vi "Property Dialog.vi"(6 "Control Ref Queue":T12, 7 "Multiplot Representation":T13, 8 "error in (no error)":errorcluster, 11 "2D Compass.lvclass in":refnum<class "2D Compass.lvclass">) -> (0 "error out":errorcluster, 3 "2D Compass.lvclass out":refnum<class "2D Compass.lvclass">, 4 "Cancel?":bool)   [LabVIEW 2020, in "2D Compass.lvclass"]
uses:
  <vilib>/Math Plots/2D Math Plots/2D Compass/2D Compass/2D Compass.lvclass
  e:/builds/penguin/labview/branches/2020/dev/dist/vi.lib/Math Plots/2D Math Plots/2D Plot/2D Plot/2D Plot.lvclass
  <vilib>/Math Plots/2D Math Plots/2D Plot/Action String/2DMathPlot Ctrl Act Queue.ctl
  <vilib>/Math Plots/2D Math Plots/2D Plot/Action String/2DMathPlot Ctrl Act Cluster.ctl
  <vilib>/Math Plots/2D Math Plots/2D Plot/Action String/2DMathPlot State Class.ctl
  <vilib>/Math Plots/2D Math Plots/2D Plot/2D Plot/Typedef/Graph General Property.ctl
  <vilib>/Math Plots/2D Math Plots/2D Compass/2D Compass/Typedef/2D Compass Property Cluster.ctl
  <vilib>/Math Plots/2D Math Plots/2D Plot/2D Plot/Typedef/Plot Property Array.ctl
  <vilib>/Math Plots/2D Math Plots/2D Plot/2D Plot/Typedef/Plot Property.ctl
  <vilib>/Math Plots/2D Math Plots/2D Compass/2D Compass/Typedef/2D Compass Property Array.ctl
  <vilib>/Math Plots/2D Math Plots/2D Compass/2D Compass/Typedef/2D Compass Property.ctl
  <vilib>/Math Plots/2D Math Plots/2D Plot/2D Plot/Typedef/Scale Cluster.ctl
  <vilib>/Utility/miscctls.llb/LVOffsetAndMultiplierTypeDef.ctl
  <vilib>/Math Plots/2D Math Plots/2D Plot/2D Plot/Typedef/Cursor Property.ctl
  <vilib>/Utility/miscctls.llb/LVCursorListTypeDef.ctl
  <vilib>/Math Plots/2D Math Plots/2D Plot/2D Plot/Typedef/Multiplot Representation.ctl
  <vilib>/Math Plots/2D Math Plots/2D Plot/2D Plot/Typedef/Plot Representation.ctl
  <vilib>/Math Plots/2D Math Plots/2D Plot/2D Plot/Typedef/Range Cluster.ctl
  <vilib>/Math Plots/2D Math Plots/2D Plot/2D Plot/Typedef/Temp Graph Data Action.ctl
  <vilib>/Math Plots/2D Math Plots/2D Plot/2D Plot/Typedef/Temp Graph State.ctl
  <vilib>/Math Plots/2D Math Plots/2D Compass/2D Compass/2D Compass.lvclass/2D Compass.ctl
  <vilib>/Math Plots/2D Math Plots/2D Plot/2D Plot/2D Plot.lvclass
panel:
  in  "Cursor Property":T1
  in  "Scales Array":T3[](array[typedef])
  in  "Compass Property":T5
  in  "Format String":string[](array[string])
  in  "Graph General":T10
  in  "Dialog Tab":enum32{"UI", "Input & Output"}(tab)
  in  "Help":bool
  in  "Cancel":bool
  in  "OK":bool
  in  "Page Tab":T11(tab)
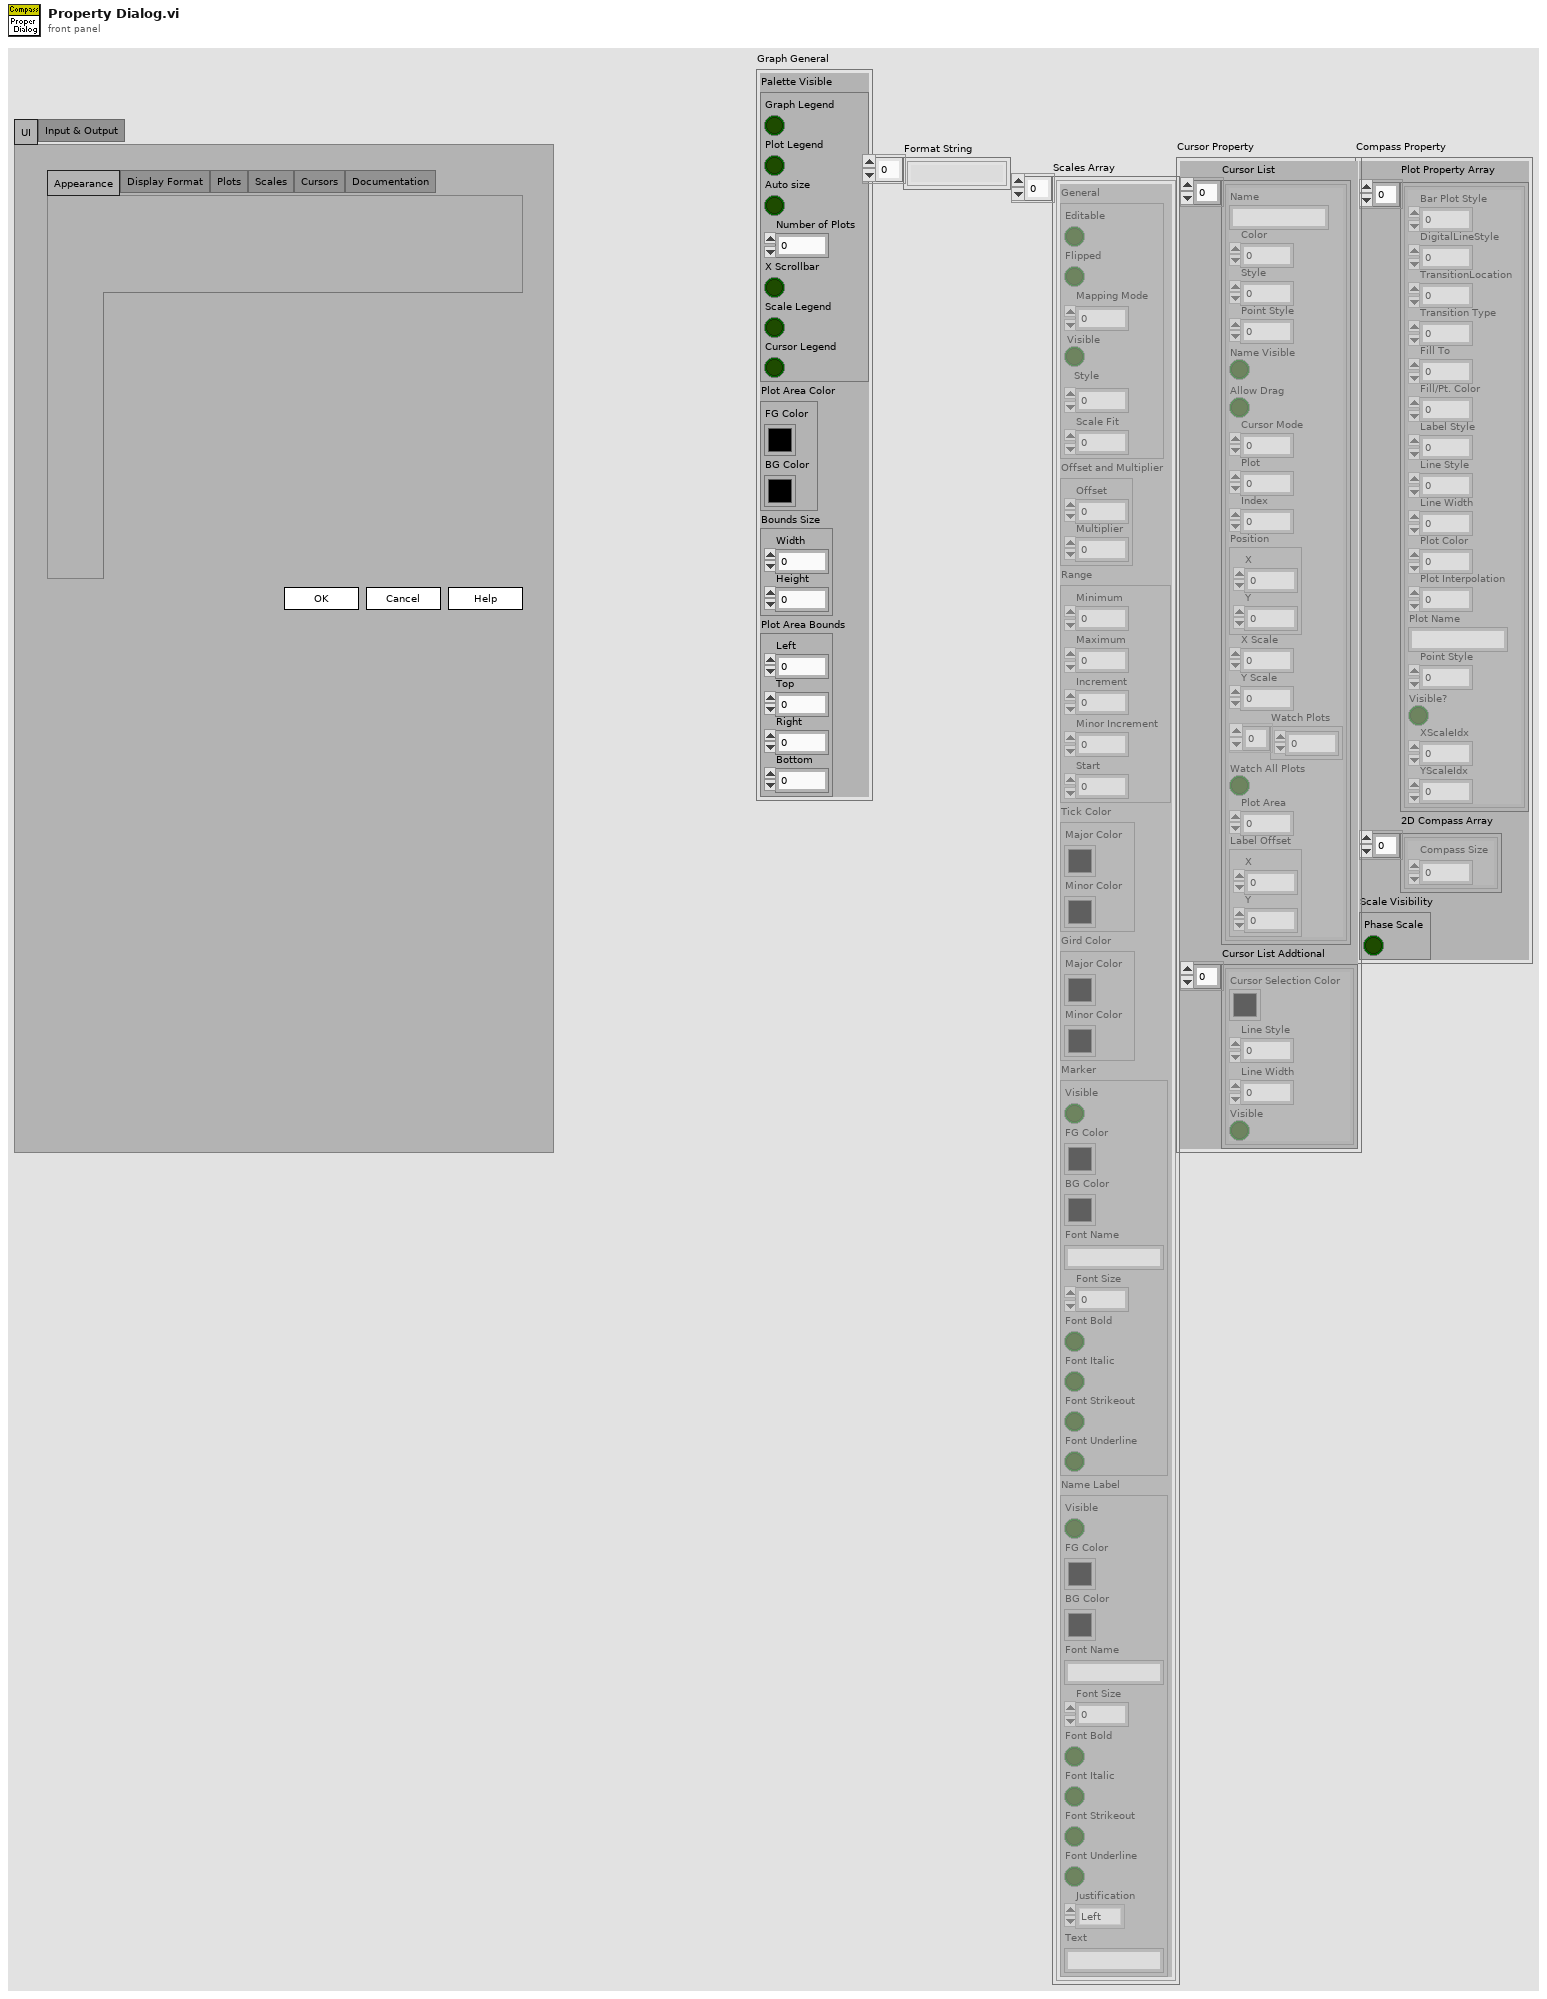
[diagram p1: front panel]
types:
  T1 = typedef "2D Plot.lvclass/Cursor Property.ctl" = cluster{"Cursor List":T2, "Cursor List Addtional":cluster{"Cursor Selection Color":u32, "Line Style":u8, "Line Width":u8, "Visible":bool}[]}
  T2 = typedef "LVCursorListTypeDef.ctl" = cluster{"Name":string, "Color":u32, "Style":u8, "Point Style":u8, "Name Visible":bool, "Allow Drag":bool, "Cursor Mode":u32, "Plot":i32, "Index":i32, "Position":cluster{"X":dbl, "Y":dbl}, "X Scale":u32, "Y Scale":u32, "Watch Plots":i32[], "Watch All Plots":bool, "Plot Area":i32, "Label Offset":cluster{"X":dbl, "Y":dbl}}[]
  T3 = typedef "2D Plot.lvclass/Scale Cluster.ctl" = cluster{"General":cluster{"Editable":bool, "Flipped":bool, "Mapping Mode":u8, "Visible":bool, "Style":u8, "Scale Fit":u8}, "Offset and Multiplier":T4, "Range":cluster{"Minimum":dbl, "Maximum":dbl, "Increment":dbl, "Minor Increment":dbl, "Start":dbl}, "Tick Color":cluster{"Major Color":u32, "Minor Color":u32}, "Gird Color":cluster{"Major Color":u32, "Minor Color":u32}, "Marker":cluster{"Visible":bool, "FG Color":u32, "BG Color":u32, "Font Name":string, "Font Size":u32, "Font Bold":bool, "Font Italic":bool, "Font Strikeout":bool, "Font Underline":bool}, "Name Label":cluster{"Visible":bool, "FG Color":u32, "BG Color":u32, "Font Name":string, "Font Size":u32, "Font Bold":bool, "Font Italic":bool, "Font Strikeout":bool, "Font Underline":bool, "Justification":enum16{"Left", "Center", "Right"}, "Text":string}}
  T4 = typedef "LVOffsetAndMultiplierTypeDef.ctl" = cluster{"Offset":dbl, "Multiplier":dbl}
  T5 = typedef "2D Compass.lvclass/2D Compass Property Cluster.ctl" = cluster{"Plot Property Array":T6, "2D Compass Array":T8, "Scale Visibility":cluster{"Phase Scale":bool}}
  T6 = typedef "2D Plot.lvclass/Plot Property Array.ctl" = T7[]
  T7 = typedef "2D Plot.lvclass/Plot Property.ctl" = cluster{"Bar Plot Style":u8, "DigitalLineStyle":u8, "TransitionLocation":u8, "Transition Type":u8, "Fill To":i16, "Fill/Pt. Color":u32, "Label Style":u8, "Line Style":u8, "Line Width":u8, "Plot Color":u32, "Plot Interpolation":u8, "Plot Name":string, "Point Style":u8, "Visible?":bool, "XScaleIdx":u32, "YScaleIdx":u32}
  T8 = typedef "2D Compass.lvclass/2D Compass Property Array.ctl" = T9[]
  T9 = typedef "2D Compass.lvclass/2D Compass Property.ctl" = cluster{"Compass Size":dbl}
  T10 = typedef "2D Plot.lvclass/Graph General Property.ctl" = cluster{"Palette Visible":cluster{"Graph Legend":bool, "Plot Legend":bool, "Auto size":bool, "Number of Plots":u32, "X Scrollbar":bool, "Scale Legend":bool, "Cursor Legend":bool}, "Plot Area Color":cluster{"FG Color":u32, "BG Color":u32}, "Bounds Size":cluster{"Width":u32, "Height":u32}, "Plot Area Bounds":cluster{"Left":i16, "Top":i16, "Right":i16, "Bottom":i16}}
  T11 = enum32{"Appearance", "Display Format", "Plots", "Scales", "Cursors", "Documentation"}
  T12 = typedef "2DMathPlot Ctrl Act Queue.ctl" = refnum<queue>
  T13 = typedef "2D Plot.lvclass/Multiplot Representation.ctl" = cluster{"Plot Representation Array":T14[], "Max Range":T15}
  T14 = typedef "2D Plot.lvclass/Plot Representation.ctl" = cluster{"Plot Range":T15, "Vertex Cluster":cluster{"Vertex X Array":dbl[], "Vertex Y Array":dbl[]}, "Base Cluster":cluster{"Base X Array":dbl[], "Base Y Array":dbl[]}}
  T15 = typedef "2D Plot.lvclass/Range Cluster.ctl" = cluster{"X Range":cluster{"Max X":dbl, "Min X":dbl}, "Y Range":cluster{"Max Y":dbl, "Min Y":dbl}}
  T16 = typedef "2D Plot.lvclass/Temp Graph State.ctl" = enum16{"Create", "Update Graph", "Update Property Only", "Get Plot Name", "Get Axis Name", "Destory"}
  T17 = typedef "2D Plot.lvclass/Temp Graph Data Action.ctl" = enum16{"Data Cluster", "Property Class", "Control Queue"}
  T18 = typedef "2D Plot.lvclass/Property Cluster.ctl" = cluster{"Graph General":T10, "Format Property":string[], "Scale Array":T19, "Cursor Property":T1, "Annotation List":T20, "Active Cursor":i32, "Active Plot":i32}
  T19 = typedef "2D Plot.lvclass/Scale Array.ctl" = T3[]
  T20 = typedef "LVAnnotationListTypeDef.ctl" = cluster{"Name":string, "Color":u32, "Style":u8, "Point Style":u8, "Name Visible":bool, "Allow Drag":bool, "Annotation Mode":u32, "Plot":i32, "Index":i32, "Position":cluster{"X":dbl, "Y":dbl}, "X Scale":u32, "Y Scale":u32, "Show Arrow":bool, "Lock Name":bool, "Plot Area":i32, "Label Offset":cluster{"X":dbl, "Y":dbl}}[]
  T21 = typedef "2DMathPlot Ctrl Act Cluster.ctl" = cluster{"Plot Area Ref":refnum<vi>, "Z Axis Ref":refnum<vi>, "Legend Ref":refnum<vi>, "XControl Ref":refnum<vi>, "Facade Ref":refnum<vi>, "Display State Change Class":T22}
  T22 = typedef "2DMathPlot State Class.ctl" = enum16{"Update All (Undo)", "Update General", "Update Appearance", "Update Format", "Update Scale", "Update Marker", "Update Cursor", "None"}
  T23 = cluster{"Plot Property Array":T6, "2D Compass Array":T8, "Scale Visibility":cluster{"Phase Scale":bool}}
  T24 = enum8{"Enabled", "Disabled", "Disabled and Grayed Out"}
  T25 = enum32{"Bad", "Idle", "Run top level", "Running"}[]
  T26 = enum32{"Bad", "Idle", "Run top level", "Running"}
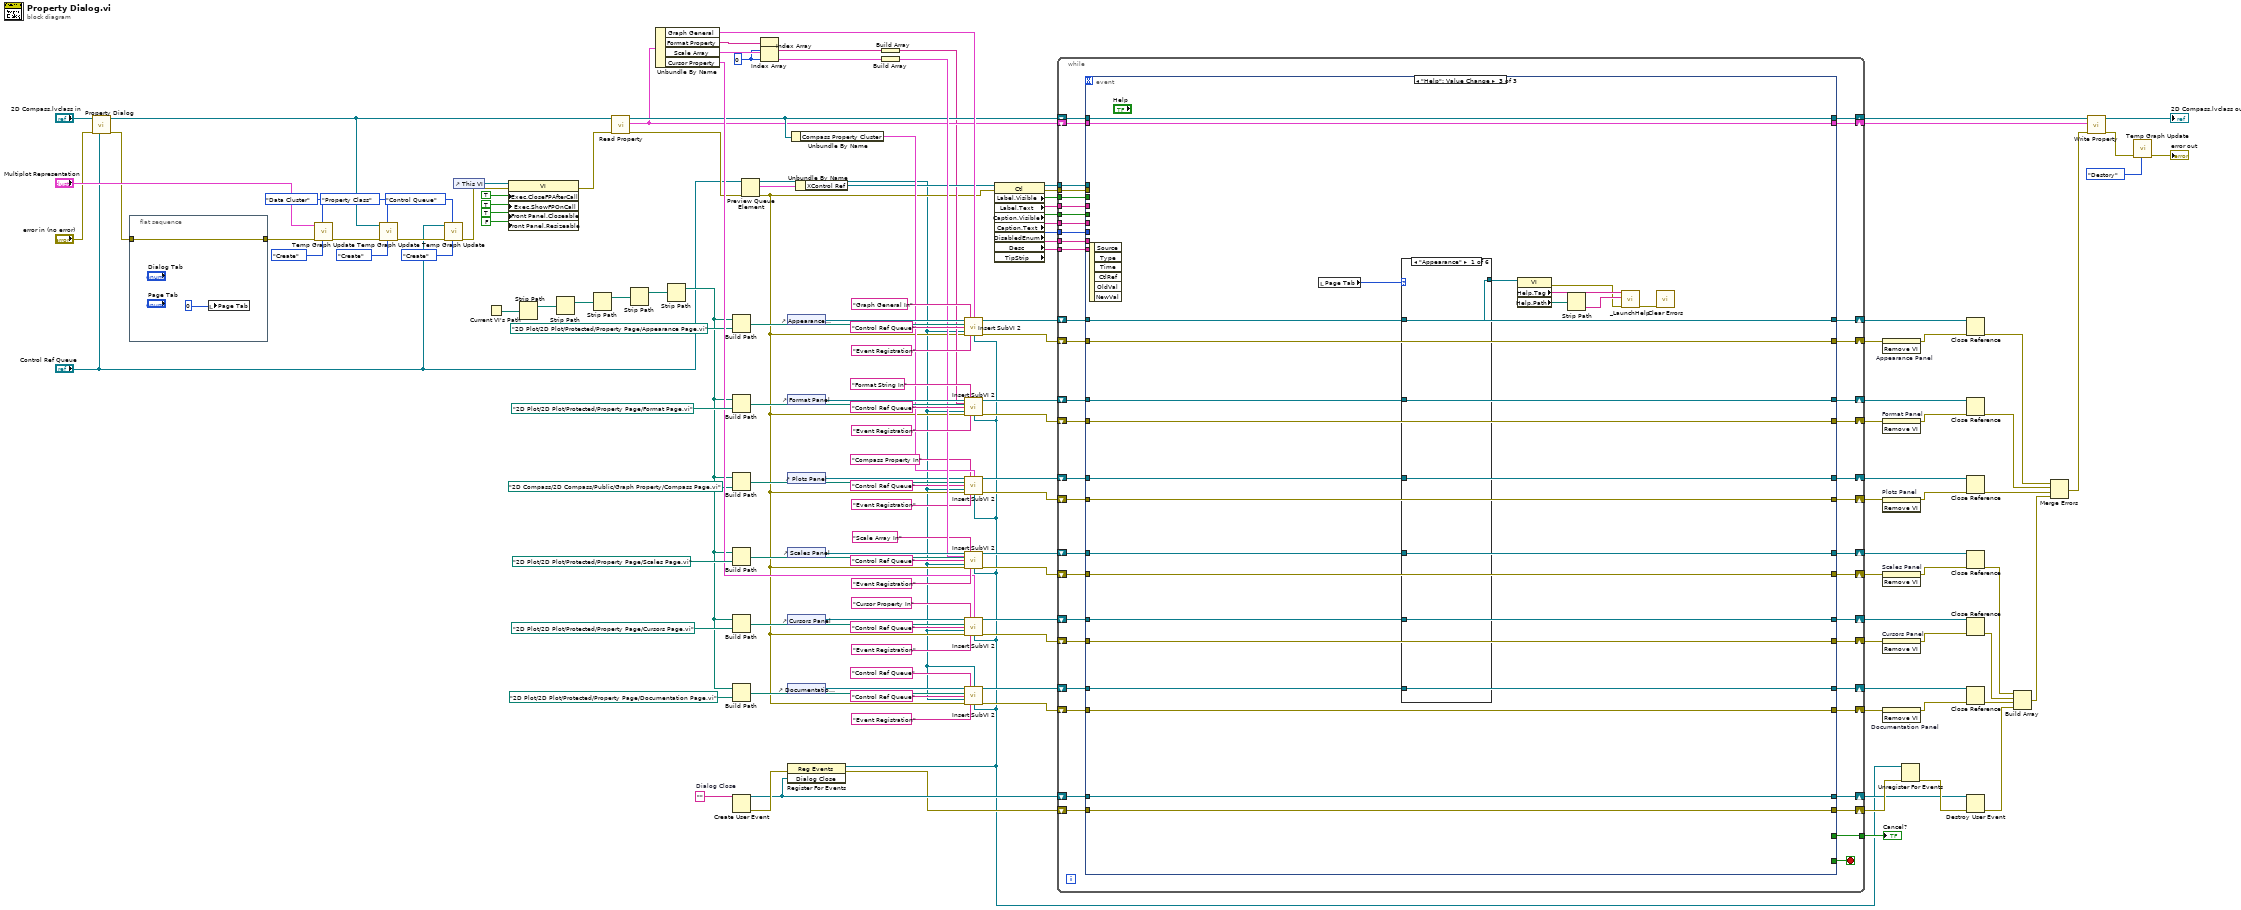
[diagram p0: block diagram]
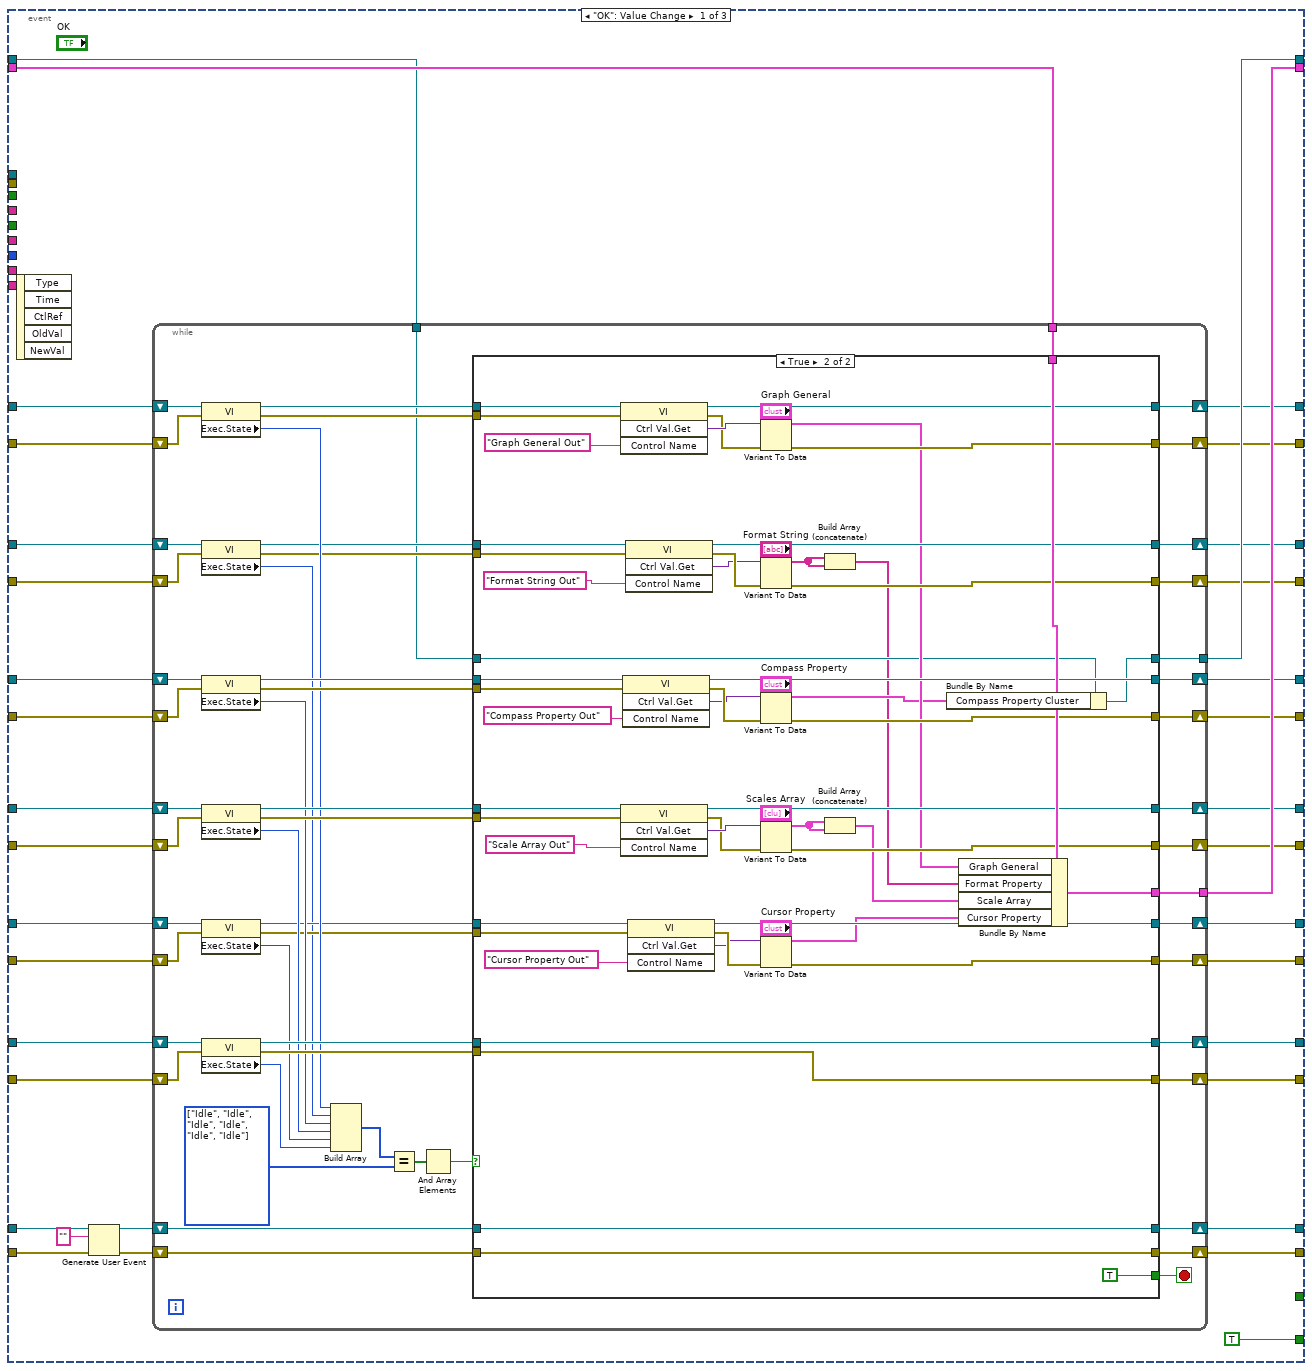
[diagram p2: hidden frame]
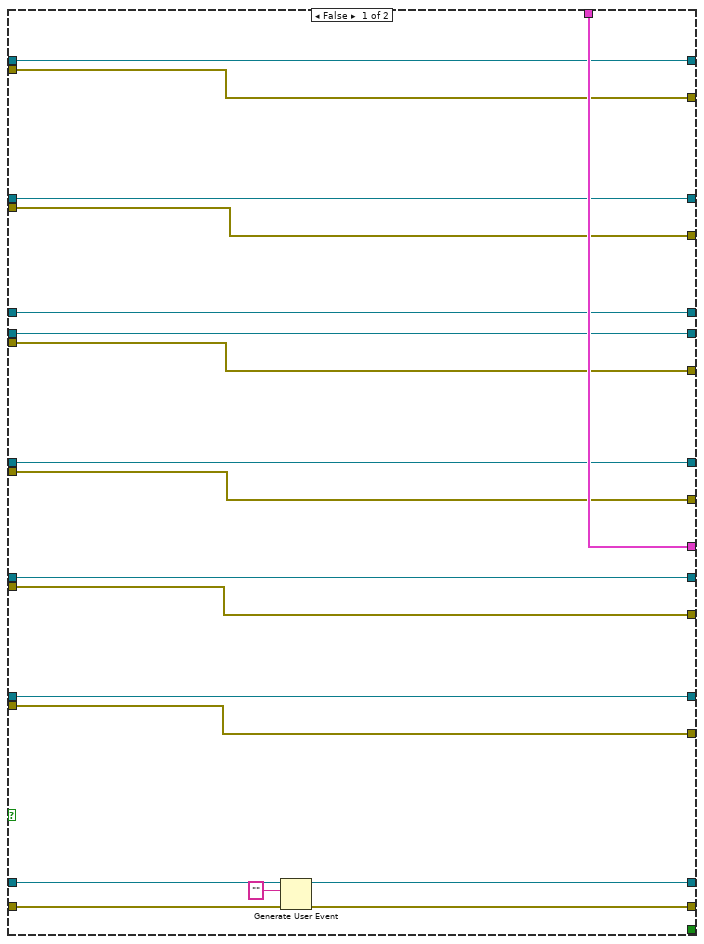
[diagram p3: hidden frame]
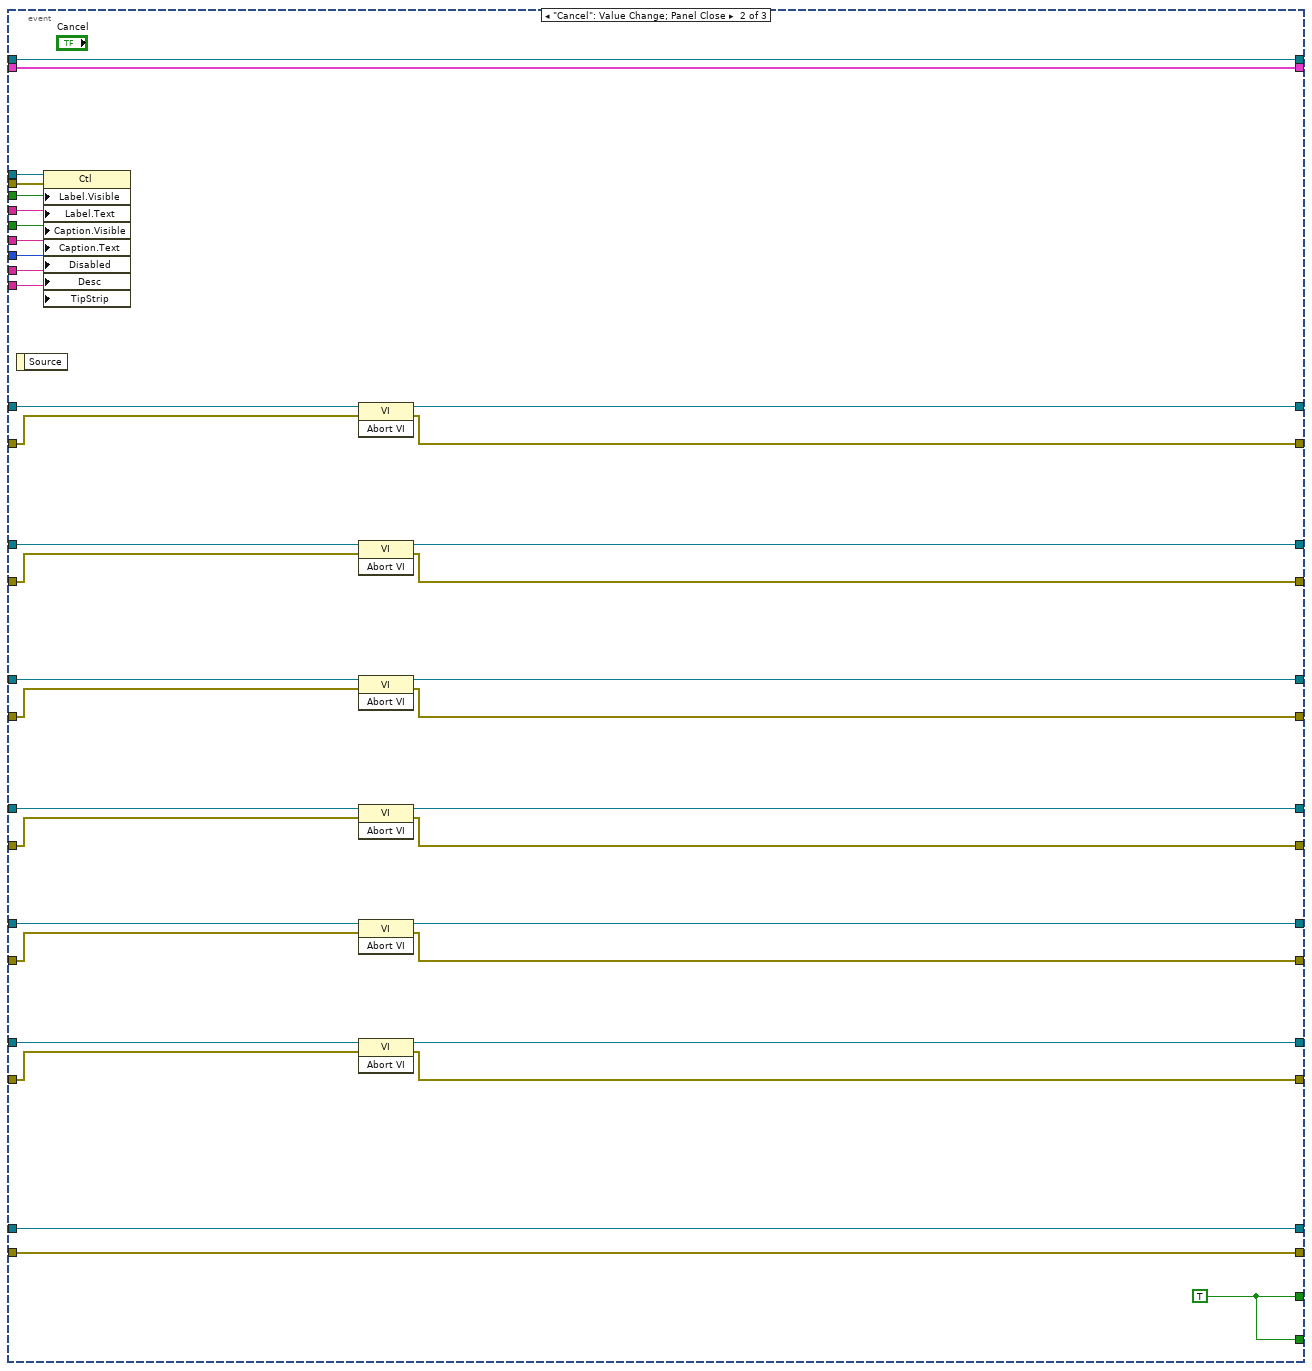
[diagram p4: hidden frame]
diagram:
  w30 = 0 ("index")
  w128 = ""  # Dialog Close
  n1 = call-parent "Property Dialog.vi"("Control Ref Queue"="Control Ref Queue", "error in (no error)"="error in (no error)", "2D Plot.lvclass in"="2D Compass.lvclass in") -> ("error out"=w2:errorcluster, "2D Plot.lvclass out"=w4:refnum<class "2D Compass.lvclass">)  [unwired: 1 in, 6 out]
  n2 = flat-sequence {
    tunnel: w2 -> [w145]
    tunnel: [w145] -> w27
    frame #0 {
      n3 = local write "Page Tab"(u32 0) -> ()
    }
  }
  n4 = call <vilib>:"Temp Graph Update.vi"("State"=Temp_Graph_State."Create", "Data Name"=Temp_Graph_Data_Action."Data Cluster", "error in (no error)"=w27, "Property In"="Multiplot Representation") -> ("error out"=w26:errorcluster)  [unwired: 1 in, 6 out]
  n5 = call <vilib>:"Temp Graph Update.vi"("State"=Temp_Graph_State."Create", "Data Name"=Temp_Graph_Data_Action."Property Class", "error in (no error)"=w26, "Property In"=w4) -> ("error out"=w25:errorcluster)  [unwired: 1 in, 6 out]
  n6 = call <vilib>:"Temp Graph Update.vi"("State"=Temp_Graph_State."Create", "Data Name"=Temp_Graph_Data_Action."Control Queue", "error in (no error)"=w25, "Property In"="Control Ref Queue") -> ("error out"=w18:errorcluster)  [unwired: 1 in, 6 out]
  n7 = control-ref of="This VI"() -> (w144:refnum<vi>)
  n8 = Current VI's Path() -> (path=w137:path)
  n9 = property class="VI"(reference=w144, error in=w18, "Exec.CloseFPAfterCall"=TRUE ("Execution:Close After Call"), "Exec.ShowFPOnCall"=TRUE ("Execution:Show Front Panel On Call"), "Front Panel.Closeable"=TRUE ("Front Panel Window:Closeable"), "Front Panel.Resizeable"=FALSE ("Front Panel Window:Resizeable")) -> (error out=w135:errorcluster)  [unwired: 1 out]
  n10 = Strip Path(path=w137) -> (stripped path=w138:path)  [unwired: 1 out]
  n11 = Strip Path(path=w138) -> (stripped path=w139:path)  [unwired: 1 out]
  n12 = Strip Path(path=w139) -> (stripped path=w136:path)  [unwired: 1 out]
  n13 = call <vilib>:"Read Property.vi"("error in (no error)"=w135, "2D Plot.lvclass in"=w4) -> ("error out"=w43:errorcluster, "XY Graph Property Cluster"=w91:T18, "2D Plot.lvclass out"=w92:refnum<class "2D Compass.lvclass">)  [unwired: 7 out]
  n14 = Strip Path(path=w136) -> (stripped path=w7:path)  [unwired: 1 out]
  n15 = Unbundle By Name(w91) -> ("Graph General"=w131:T10, "Format Property"=w29:string[], "Scale Array"=w31:T19, "Cursor Property"=w111:T1)
  n16 = Strip Path(path=w7) -> (stripped path=w6:path)  [unwired: 1 out]
  n17 = Build Path(base path=w6, name or relative path=path "2D Plot/2D Plot/Protected/Property Page/Appearance Page.vi") -> (appended path=w134:path)
  n18 = Build Path(base path=w6, name or relative path=path "2D Plot/2D Plot/Protected/Property Page/Format Page.vi") -> (appended path=w124:path)
  n19 = Build Path(base path=w6, name or relative path=path "2D Compass/2D Compass/Public/Graph Property/Compass Page.vi") -> (appended path=w95:path)
  n20 = Build Path(base path=w6, name or relative path=path "2D Plot/2D Plot/Protected/Property Page/Scales Page.vi") -> (appended path=w117:path)
  n21 = Build Path(base path=w6, name or relative path=path "2D Plot/2D Plot/Protected/Property Page/Cursors Page.vi") -> (appended path=w106:path)
  n22 = Build Path(base path=w6, name or relative path=path "2D Plot/2D Plot/Protected/Property Page/Documentation Page.vi") -> (appended path=w97:path)
  n23 = Create User Event(user event datatype=w128) -> (user event=w78:refnum<user-event>, error out=w129:errorcluster)  [unwired: 1 in]
  n24 = Preview Queue Element(queue="Control Ref Queue", error in (no error)=w43) -> (queue out=w11:T12, element=w42:T21, error out=w12:errorcluster)  [unwired: 2 out]
  n25 = Index Array(array=w29, index=w30) -> (element=w28:string)
  n26 = Index Array(array=w31, index=w30) -> (element=w120:T3)
  n27 = control-ref of="Appearance Panel"() -> (w133:refnum<vi>)
  n28 = control-ref of="Format Panel"() -> (w125:refnum<vi>)
  n29 = control-ref of="Plots Panel"() -> (w102:refnum<vi>)
  n30 = control-ref of="Scales Panel"() -> (w119:refnum<vi>)
  n31 = control-ref of="Cursors Panel"() -> (w108:refnum<vi>)
  n32 = control-ref of="Documentation Panel"() -> (w105:refnum<vi>)
  n33 = register-events(error in=w129, w78) -> (reference out=w10:refnum<event-registration>, error out=w77:errorcluster)  [unwired: 1 in]
  n34 = Unbundle By Name(w92) -> ("Compass Property Cluster"=w99:T23)
  n35 = Unbundle By Name(w42) -> ("XControl Ref"=w41:refnum<vi>)
  n36 = Build Array(w28) -> (w13:string[])
  n37 = Build Array(w120) -> (w114:T3[])
  n38 = call <vilib>:"Insert SubVI 2.vi"("Sub Panel Ref"=w133, "Label 1"="Graph General In", "Value 1"=w131, "VI Path"=w134, "Label 3"="Control Ref Queue" ("Label 1"), "Value 3"=w11, "error in (no error)"=w12, "Label 2"="Event Registration", "Value 2"=w10) -> ("vi reference"=w90:refnum<vi>, "error out"=w84:errorcluster)  [unwired: 5 out]
  n39 = call <vilib>:"Insert SubVI 2.vi"("Sub Panel Ref"=w125, "Label 1"="Format String In" ("Label 2"), "Value 1"=w13, "VI Path"=w124, "Label 3"="Control Ref Queue" ("Label 1"), "Value 3"=w11, "error in (no error)"=w12, "Label 2"="Event Registration", "Value 2"=w10) -> ("vi reference"=w89:refnum<vi>, "error out"=w83:errorcluster)  [unwired: 5 out]
  n40 = call <vilib>:"Insert SubVI 2.vi"("Sub Panel Ref"=w102, "Label 1"="Compass Property In", "Value 1"=w99, "VI Path"=w95, "Label 3"="Control Ref Queue" ("Label 1"), "Value 3"=w11, "error in (no error)"=w12, "Label 2"="Event Registration", "Value 2"=w10) -> ("vi reference"=w88:refnum<vi>, "error out"=w82:errorcluster)  [unwired: 5 out]
  n41 = call <vilib>:"Insert SubVI 2.vi"("Sub Panel Ref"=w119, "Label 1"="Scale Array In", "Value 1"=w114, "VI Path"=w117, "Label 3"="Control Ref Queue" ("Label 1"), "Value 3"=w11, "error in (no error)"=w12, "Label 2"="Event Registration", "Value 2"=w10) -> ("vi reference"=w87:refnum<vi>, "error out"=w81:errorcluster)  [unwired: 5 out]
  n42 = call <vilib>:"Insert SubVI 2.vi"("Sub Panel Ref"=w108, "Label 1"="Cursor Property In", "Value 1"=w111, "VI Path"=w106, "Label 3"="Control Ref Queue" ("Label 1"), "Value 3"=w11, "error in (no error)"=w12, "Label 2"="Event Registration", "Value 2"=w10) -> ("vi reference"=w86:refnum<vi>, "error out"=w80:errorcluster)  [unwired: 5 out]
  n43 = call <vilib>:"Insert SubVI 2.vi"("Sub Panel Ref"=w105, "Label 1"="Control Ref Queue", "Value 1"=w11, "VI Path"=w97, "Label 3"="Control Ref Queue" ("Label 1"), "Value 3"=w11, "error in (no error)"=w12, "Label 2"="Event Registration", "Value 2"=w10) -> ("vi reference"=w85:refnum<vi>, "error out"=w79:errorcluster)  [unwired: 5 out]
  n44 = property class="Ctl"(reference=w41, error in=w12) -> (reference out=w40:refnum<vi>, error out=w39:errorcluster, "Label.Visible"=w38:bool, "Label.Text"=w37:string, "Caption.Visible"=w36:bool, "Caption.Text"=w35:string, "DisabledEnum"=w34:T24, "Desc"=w33:string, "TipStrip"=w32:string)
  n45 = while {
    shift-right: [w173] -> w74
    shift-left: w92 -> [w189]
    shift-right: [w172] -> w75
    shift-left: w91 -> [w188]
    shift-right: [w171] -> w65
    shift-left: w84 -> [w181]
    shift-right: [w170] -> w63
    shift-left: w83 -> [w180]
    shift-right: [w169] -> w57
    shift-left: w82 -> [w179]
    shift-right: [w168] -> w54
    shift-left: w81 -> [w178]
    shift-right: [w167] -> w53
    shift-left: w80 -> [w177]
    shift-right: [w166] -> w49
    shift-left: w79 -> [w176]
    shift-right: [w165] -> w46
    shift-left: w77 -> [w174]
    shift-right: [w158] -> w44
    shift-left: w78 -> [w175]
    shift-right: [w159] -> w48
    shift-left: w85 -> [w182]
    shift-right: [w160] -> w52
    shift-left: w86 -> [w183]
    shift-right: [w161] -> w56
    shift-left: w87 -> [w184]
    shift-right: [w162] -> w58
    shift-left: w88 -> [w185]
    shift-right: [w163] -> w61
    shift-left: w89 -> [w186]
    shift-right: [w164] -> w66
    shift-left: w90 -> [w187]
    tunnel: [w156] -> w76
    tunnel: w40 -> [w155]
    tunnel: w39 -> [w154]
    tunnel: w38 -> [w153]
    tunnel: w37 -> [w152]
    tunnel: w36 -> [w151]
    tunnel: w35 -> [w150]
    tunnel: w34 -> [w149]
    tunnel: w33 -> [w148]
    tunnel: w32 -> [w147]
    stop <- w157 stop-if-true
    n46 = event shown="[2] \"Help\": Value Change" {
      selector: _ -> [_ _ _]
      dyn-events: _ -> [_ _ _]
      timeout: _ -> [_ _ _]
      tunnel: w189 -> [w207 w366 w407]
      tunnel: w188 -> [w208 w367 w408]
      tunnel: w187 -> [w225 w393 w400]
      tunnel: w186 -> [w224 w389 w399]
      tunnel: w185 -> [w223 w387 w398]
      tunnel: w184 -> [w222 w385 w397]
      tunnel: w183 -> [w221 w383 w396]
      tunnel: w182 -> [w220 w381 w395]
      tunnel: w181 -> [w219 w392 w416]
      tunnel: w180 -> [w218 w388 w415]
      tunnel: w179 -> [w217 w386 w414]
      tunnel: w178 -> [w216 w384 w413]
      tunnel: w177 -> [w215 w382 w412]
      tunnel: w176 -> [w214 w380 w411]
      tunnel: w175 -> [w210 w369 w409]
      tunnel: w174 -> [w211 w368 w410]
      tunnel: [w206 w366 w407] -> w173
      tunnel: [w205 w367 w408] -> w172
      tunnel: [w204 w390 w416] -> w171
      tunnel: [w203 w378 w415] -> w170
      tunnel: [w190 w376 w414] -> w169
      tunnel: [w191 w374 w413] -> w168
      tunnel: [w202 w372 w412] -> w167
      tunnel: [w201 w370 w411] -> w166
      tunnel: [w200 w368 w410] -> w165
      tunnel: [w199 w391 w400] -> w164
      tunnel: [w198 w379 w399] -> w163
      tunnel: [w197 w377 w398] -> w162
      tunnel: [w196 w375 w397] -> w161
      tunnel: [w195 w373 w396] -> w160
      tunnel: [w194 w371 w395] -> w159
      tunnel: [w192 w369 w409] -> w158
      tunnel: [TRUE w356 _] -> w157
      tunnel: [_ w356 _] -> w156
      tunnel: w155 -> [_ w365 _]
      tunnel: w154 -> [_ w364 _]
      tunnel: w153 -> [_ w363 _]
      tunnel: w152 -> [_ w362 _]
      tunnel: w151 -> [_ w361 _]
      tunnel: w150 -> [_ w360 _]
      tunnel: w149 -> [_ w359 _]
      tunnel: w148 -> [_ w358 _]
      tunnel: w147 -> [_ w357 _]
      event "OK": Value Change {
        n47 = event-data() -> ()  [unwired: 6 out]
        n48 = Generate User Event(user event=w210, event data cluster="" ("event data"), error in=w211) -> (user event out=w209:refnum<user-event>, error out=w212:errorcluster)  [unwired: 1 in]
        n49 = while {
          tunnel: w208 -> [w280]
          tunnel: [w279] -> w205
          shift-right: [w246] -> w192
          shift-left: w209 -> [w247]
          shift-right: [w230] -> w200
          shift-left: w212 -> [w239]
          tunnel: w207 -> [w229]
          tunnel: [w228] -> w206
          shift-right: [w257] -> w201
          shift-left: w214 -> [w253]
          shift-right: [w256] -> w194
          shift-left: w220 -> [w252]
          shift-right: [w233] -> w195
          shift-left: w221 -> [w238]
          shift-right: [w234] -> w202
          shift-left: w215 -> [w237]
          shift-right: [w227] -> w191
          shift-left: w216 -> [w261]
          shift-right: [w258] -> w196
          shift-left: w222 -> [w262]
          shift-right: [w264] -> w197
          shift-left: w223 -> [w267]
          shift-right: [w226] -> w190
          shift-left: w217 -> [w263]
          shift-right: [w241] -> w198
          shift-left: w224 -> [w244]
          shift-right: [w240] -> w203
          shift-left: w218 -> [w245]
          shift-right: [w278] -> w199
          shift-left: w225 -> [w276]
          shift-right: [w277] -> w204
          shift-left: w219 -> [w274]
          stop <- w268 stop-if-true
          w271 = T25 [enum."Idle", enum."Idle", enum."Idle", enum."Idle", enum."Idle", enum."Idle"] items=["Bad", "Idle", "Run top level", "Running"]
          n50 = property class="VI"(reference=w276, error in=w274) -> (reference out=w275:refnum<vi>, error out=w273:errorcluster, "Exec.State"=w251:T26)
          n51 = property class="VI"(reference=w244, error in=w245) -> (reference out=w243:refnum<vi>, error out=w242:errorcluster, "Exec.State"=w232:T26)
          n52 = property class="VI"(reference=w267, error in=w263) -> (reference out=w266:refnum<vi>, error out=w265:errorcluster, "Exec.State"=w250:T26)
          n53 = property class="VI"(reference=w262, error in=w261) -> (reference out=w260:refnum<vi>, error out=w259:errorcluster, "Exec.State"=w249:T26)
          n54 = property class="VI"(reference=w238, error in=w237) -> (reference out=w236:refnum<vi>, error out=w235:errorcluster, "Exec.State"=w231:T26)
          n55 = property class="VI"(reference=w252, error in=w253) -> (reference out=w254:refnum<vi>, error out=w255:errorcluster, "Exec.State"=w248:T26)
          n56 = Build Array(w251, w232, w250, w249, w231, w248) -> (w272:T25)
          n57 = Equal?(x=w272, y=w271) -> (x = y?=w270:bool[])
          n58 = And Array Elements(Boolean array=w270) -> (logical AND=w269:bool)
          n59 = case shown="True" w269 {
            tunnel: w280 -> [w299 w355]
            tunnel: [w299 w354] -> w279
            tunnel: [w298 w350] -> w278
            tunnel: [w297 w349] -> w277
            tunnel: w275 -> [w298 w348]
            tunnel: w273 -> [w297 w347]
            tunnel: [_ TRUE] -> w268
            tunnel: w266 -> [w295 w341]
            tunnel: w265 -> [w296 w342]
            tunnel: [w296 w340] -> w226
            tunnel: [w295 w339] -> w264
            tunnel: w260 -> [w293 w335]
            tunnel: w259 -> [w294 w334]
            tunnel: [w293 w333] -> w258
            tunnel: [w294 w332] -> w227
            tunnel: w254 -> [w292 w305]
            tunnel: w255 -> [w291 w304]
            tunnel: [w292 w305] -> w256
            tunnel: [w291 w304] -> w257
            tunnel: w247 -> [w290 w331]
            tunnel: [w289 w331] -> w246
            tunnel: w243 -> [w287 w327]
            tunnel: w242 -> [w286 w326]
            tunnel: [w287 w325] -> w241
            tunnel: [w286 w324] -> w240
            tunnel: w239 -> [w285 w323]
            tunnel: [w284 w323] -> w230
            tunnel: w236 -> [w283 w319]
            tunnel: w235 -> [w282 w318]
            tunnel: [w282 w317] -> w234
            tunnel: [w283 w316] -> w233
            tunnel: w229 -> [w281 w312]
            tunnel: [w281 w306] -> w228
            frame False {
              n60 = Generate User Event(user event=w290, event data cluster="" ("event data"), error in=w285) -> (user event out=w289:refnum<user-event>, error out=w284:errorcluster)  [unwired: 1 in]
            }
            frame True {
              n61 = invoke class="VI" method="Ctrl Val.Get"(reference=w348, error in=w347, "Control Name"="Graph General Out") -> (reference out=w350:refnum<vi>, error out=w351:errorcluster, "Get Control Value Variant"=w352:variant)  [unwired: 1 in, 1 out]
              n62 = invoke class="VI" method="Ctrl Val.Get"(reference=w335, error in=w334, "Control Name"="Scale Array Out") -> (reference out=w333:refnum<vi>, error out=w336:errorcluster, "Get Control Value Variant"=w337:variant)  [unwired: 1 in, 1 out]
              n63 = invoke class="VI" method="Ctrl Val.Get"(reference=w341, error in=w342, "Control Name"="Compass Property Out") -> (reference out=w339:refnum<vi>, error out=w345:errorcluster, "Get Control Value Variant"=w344:variant)  [unwired: 1 in, 1 out]
              n64 = invoke class="VI" method="Ctrl Val.Get"(reference=w327, error in=w326, "Control Name"="Format String Out") -> (reference out=w325:refnum<vi>, error out=w330:errorcluster, "Get Control Value Variant"=w329:variant)  [unwired: 1 in, 1 out]
              n65 = invoke class="VI" method="Ctrl Val.Get"(reference=w319, error in=w318, "Control Name"="Cursor Property Out") -> (reference out=w316:refnum<vi>, error out=w322:errorcluster, "Get Control Value Variant"=w321:variant)  [unwired: 1 in, 1 out]
              n66 = Variant To Data(error in=w351, type="Graph General", Variant=w352) -> (data=w314:T10, error out=w349:errorcluster)
              n67 = Variant To Data(error in=w330, type="Format String", Variant=w329) -> (data=w303:string[], error out=w324:errorcluster)
              n68 = Variant To Data(error in=w345, type="Compass Property", Variant=w344) -> (data=w310:T5, error out=w340:errorcluster)
              n69 = Variant To Data(error in=w336, type="Scales Array", Variant=w337) -> (data=w301:T3[], error out=w332:errorcluster)
              n70 = Variant To Data(error in=w322, type="Cursor Property", Variant=w321) -> (data=w307:T1, error out=w317:errorcluster)
              n71 = Build Array (concatenate)(w303, w303) -> (w302:string[])
              n72 = Build Array (concatenate)(w301, w301) -> (w300:T3[])
              n73 = Bundle By Name(cluster=w312, "Compass Property Cluster"=w310) -> (w306:refnum<class "2D Compass.lvclass">)
              n74 = Bundle By Name(cluster=w355, "Graph General"=w314, "Format Property"=w302, "Scale Array"=w300, "Cursor Property"=w307) -> (w354:T18)
            }
          }
        }
      }
      event "Cancel": Value Change; Panel Close {
        w356 = TRUE
        n75 = event-data() -> ()  [unwired: 2 out]
        n76 = property class="Ctl"(reference=w365, error in=w364, "Label.Visible"=w363, "Label.Text"=w362, "Caption.Visible"=w361, "Caption.Text"=w360, "Disabled"=w359, "Desc"=w358, "TipStrip"=w357) -> ()  [unwired: 2 out]
        n77 = invoke class="VI" method="Abort VI"(reference=w393, error in=w392) -> (reference out=w391:refnum<vi>, error out=w390:errorcluster)  [unwired: 1 in, 1 out]
        n78 = invoke class="VI" method="Abort VI"(reference=w389, error in=w388) -> (reference out=w379:refnum<vi>, error out=w378:errorcluster)  [unwired: 1 in, 1 out]
        n79 = invoke class="VI" method="Abort VI"(reference=w387, error in=w386) -> (reference out=w377:refnum<vi>, error out=w376:errorcluster)  [unwired: 1 in, 1 out]
        n80 = invoke class="VI" method="Abort VI"(reference=w385, error in=w384) -> (reference out=w375:refnum<vi>, error out=w374:errorcluster)  [unwired: 1 in, 1 out]
        n81 = invoke class="VI" method="Abort VI"(reference=w383, error in=w382) -> (reference out=w373:refnum<vi>, error out=w372:errorcluster)  [unwired: 1 in, 1 out]
        n82 = invoke class="VI" method="Abort VI"(reference=w381, error in=w380) -> (reference out=w371:refnum<vi>, error out=w370:errorcluster)  [unwired: 1 in, 1 out]
      }
      event "Help": Value Change {
        n83 = event-data() -> ()  [unwired: 7 out]
        n84 = local read "Page Tab"() -> (w394:T11)
        n85 = case shown="\"Appearance\"" w394 {
          tunnel: w400 -> [w417 _ _ _ _ _]
          tunnel: [w417 w418 w419 w420 w421 w422] -> w401
          tunnel: w399 -> [_ w418 _ _ _ _]
          tunnel: w398 -> [_ _ w419 _ _ _]
          tunnel: w397 -> [_ _ _ w420 _ _]
          tunnel: w396 -> [_ _ _ _ w421 _]
          tunnel: w395 -> [_ _ _ _ _ w422]
          frame "Appearance" {
          }
          frame "Display Format" {
          }
          frame "Plots" {
          }
          frame "Scales" {
          }
          frame "Cursors" {
          }
          frame "Documentation" {
          }
        }
        n86 = property class="VI"(reference=w401) -> (error out=w403:errorcluster, "Help.Tag"=w405:string, "Help.Path"=w406:path)  [unwired: 1 in, 1 out]
        n87 = Strip Path(path=w406) -> (name=w404:string)  [unwired: 1 out]
        n88 = call <helpdir>:"_LaunchHelp.vi"("error in (no error)"=w403, "CHM or HLP filename (lvdialog.chm)"=w404, "HTML filename"=w405) -> ("error out"=w402:errorcluster)  [unwired: 4 out]
        n89 = call <vilib>:"Clear Errors.vi"("error in (no error)"=w402) -> ()  [unwired: 5 in, 2 out]
      }
    }
  }
  "Cancel?" <- w76
  n90 = invoke on="Appearance Panel" class="SubPnl" method="Remove VI"(error in=w65) -> (error out=w64:errorcluster)  [unwired: 2 in, 2 out]
  n91 = invoke on="Format Panel" class="SubPnl" method="Remove VI"(error in=w63) -> (error out=w62:errorcluster)  [unwired: 2 in, 2 out]
  n92 = invoke on="Plots Panel" class="SubPnl" method="Remove VI"(error in=w57) -> (error out=w59:errorcluster)  [unwired: 2 in, 2 out]
  n93 = invoke on="Scales Panel" class="SubPnl" method="Remove VI"(error in=w54) -> (error out=w55:errorcluster)  [unwired: 2 in, 2 out]
  n94 = invoke on="Cursors Panel" class="SubPnl" method="Remove VI"(error in=w53) -> (error out=w51:errorcluster)  [unwired: 2 in, 2 out]
  n95 = invoke on="Documentation Panel" class="SubPnl" method="Remove VI"(error in=w49) -> (error out=w50:errorcluster)  [unwired: 2 in, 2 out]
  n96 = Unregister For Events(event registration refnum=w10, error in=w46) -> (error out=w45:errorcluster)
  n97 = Close Reference(reference=w66, error in (no error)=w64) -> (error out=w60:errorcluster)
  n98 = Close Reference(reference=w61, error in (no error)=w62) -> (error out=w70:errorcluster)
  n99 = Close Reference(reference=w58, error in (no error)=w59) -> (error out=w69:errorcluster)
  n100 = Close Reference(reference=w56, error in (no error)=w55) -> (error out=w71:errorcluster)
  n101 = Close Reference(reference=w52, error in (no error)=w51) -> (error out=w72:errorcluster)
  n102 = Close Reference(reference=w48, error in (no error)=w50) -> (error out=w67:errorcluster)
  n103 = Destroy User Event(user event=w44, error in=w45) -> (error out=w9:errorcluster)
  n104 = Build Array(w71, w72, w67, w9) -> (w68:errorcluster[])
  n105 = Merge Errors(w60, w70, w69, w68) -> (w47:errorcluster)
  n106 = call <vilib>:"Write Property.vi"("error in (no error)"=w47, "XY Graph Property Cluster"=w75, "2D Plot.lvclass in"=w74) -> ("error out"=w17:errorcluster, "2D Plot.lvclass out"=→"2D Compass.lvclass out":refnum<class "2D Compass.lvclass">)  [unwired: 7 out]
  n107 = call <vilib>:"Temp Graph Update.vi"("State"=Temp_Graph_State."Destory", "error in (no error)"=w17) -> ("error out"=→"error out":errorcluster)  [unwired: 3 in, 6 out]
